vi "Frame Switch by Num.vi"(8 "error in (no error)":errorcluster, 10 "Frame Num":u32, 11 "LF2R IDE in":refnum<class "Main Panel.lvclass">) -> (0 "error out":errorcluster, 3 "LF2R IDE out":refnum<class "Main Panel.lvclass">)   [LabVIEW 2018, in "Main Panel.lvlib" / "Main Panel.lvclass"]
uses:
  Main Panel.lvclass
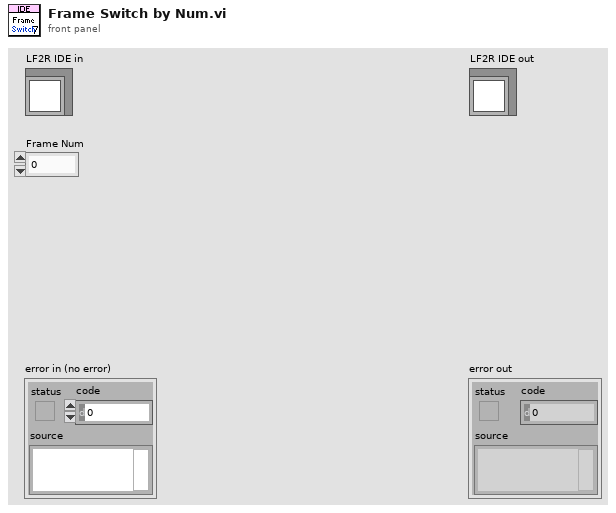
[diagram p1: front panel]
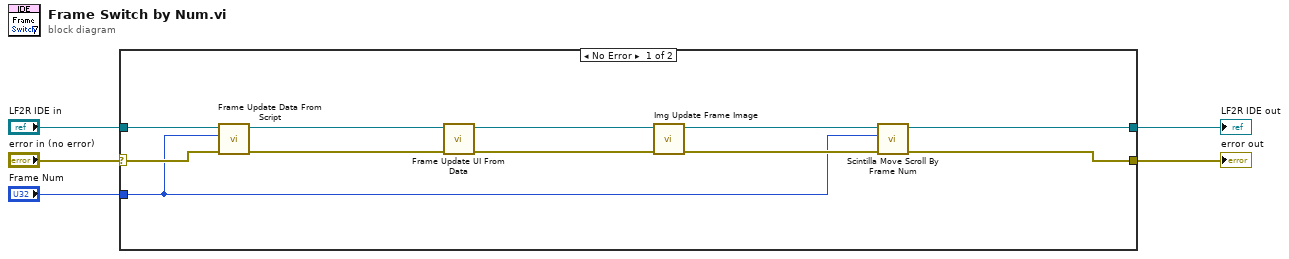
[diagram p0: block diagram]
diagram:
  n1 = case shown="No Error" "error in (no error)" {
    selector: "error in (no error)" -> [w13 w18]
    tunnel: [w11 w18] -> w3
    tunnel: [w12 w17] -> w4
    tunnel: "LF2R IDE in" -> [w16 w17]
    tunnel: "Frame Num" -> [w6 _]
    frame No Error {
      n2 = call "Frame Update Data From Script.vi"("error in (no error)"=w13, "Frame Number"=w6, "IDE simple in"=w16) -> ("error out"=w14:errorcluster, "IDE simple out"=w15:refnum<class "Main Panel.lvclass">)  [unwired: 7 in]
      n3 = call "Frame Update UI From Data.vi"("error in (no error)"=w14, "IDE simple in"=w15) -> ("error out"=w9:errorcluster, "IDE simple out"=w10:refnum<class "Main Panel.lvclass">)  [unwired: 8 in]
      n4 = call "Img Update Frame Image.vi"("error in (no error)"=w9, "LF2R IDE in"=w10) -> ("error out"=w7:errorcluster, "LF2R IDE out"=w8:refnum<class "Main Panel.lvclass">)  [unwired: 8 in]
      n5 = call "Scintilla Move Scroll By Frame Num.vi"("error in (no error)"=w7, "Frame Number"=w6, "IDE simple in"=w8) -> ("error out"=w11:errorcluster, "IDE simple out"=w12:refnum<class "Main Panel.lvclass">)  [unwired: 7 in]
    }
    frame Error {
    }
  }
  "error out" <- w3
  "LF2R IDE out" <- w4
